vi "Handle Last Ack Core.vi"(4 "error in (no error)":errorcluster, 6 "Last Ack":refnum<class "Last Ack.lvclass">, 7 "LoggingActor in":refnum<class "LoggingActor.lvclass">) -> (0 "error out":errorcluster, 3 "LoggingActor out":refnum<class "LoggingActor.lvclass">)   [LabVIEW 2022 SP3, in "LoggingActor.lvlib" / "LoggingActor.lvclass"]
doc: "(<B>Filename</B>: Actor Framework.lvlib:Actor.lvclass:Handle Last Ack Core.vi)\n\nDefines how the caller actor responds to the Last Ack message from a nested actor. The Last Ack message is the final message a nested actor sends to its caller before it shuts down. The message contains information about the final state of the nested actor.\n\nBy default, this method does nothing except return any error the nested actor sent. A descendant class may override this method to define behavior."
uses:
  LoggingActor.lvclass
  LoggingActor.lvclass/LoggingActor.ctl
  <vilib>/ActorFramework/Actor/Actor.lvclass
  Logger/Source/Logger/Logger.lvclass
  <vilib>/ActorFramework/LastAck/Last Ack.lvclass
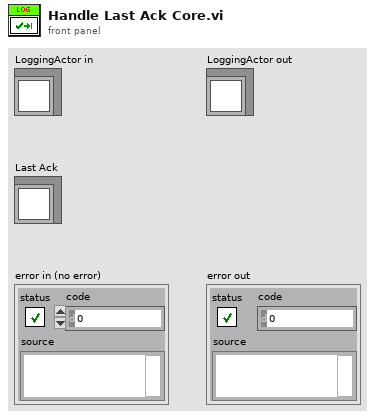
[diagram p1: front panel]
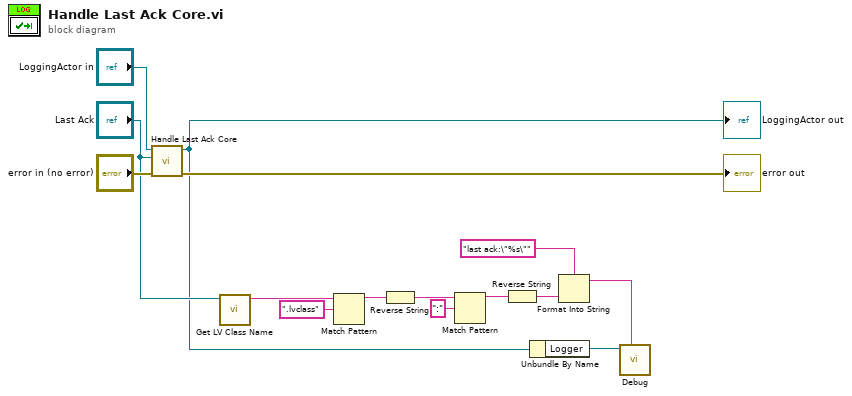
[diagram p0: block diagram]
diagram:
  n1 = call-parent "Handle Last Ack Core.vi"("error in (no error)"="error in (no error)", "Last Ack"="Last Ack", "Actor in"="LoggingActor in") -> ("error out"=→"error out":errorcluster, "Actor out"=w1:refnum<class "LoggingActor.lvclass">)  [unwired: 3 in]
  "LoggingActor out" <- w1
  n2 = call <vilib>:"Get LV Class Name.vi"("object"="Last Ack") -> ("class name"=w9:string)  [unwired: 9 in, 1 out]
  n3 = Match Pattern(string=w9, regular expression=".lvclass") -> (before substring=w8:string)  [unwired: 1 in, 3 out]
  n4 = Reverse String(1:w8) -> (0:w6:string)
  n5 = Match Pattern(string=w6, regular expression=":") -> (before substring=w5:string)  [unwired: 1 in, 3 out]
  n6 = Reverse String(1:w5) -> (0:w3:string)
  n7 = Unbundle By Name(w1) -> ("Logger"=w12:refnum<class "Logger.lvclass">)
  n8 = Format Into String(format string="last ack:\"%s\"", w3) -> (resulting string=w11:string)  [unwired: 2 in, 1 out]
  n9 = call-dynamic "Debug.vi"("Message"=w11, "Logger in"=w12) -> ()  [unwired: 6 in, 2 out]
